vi "TempConvert.vi"(1 "All type T\nTC data \nfrom module":dbl[](array[numeric])) -> (0 "Temperature (K)":dbl[](array[numeric]))   [LabVIEW 2010]
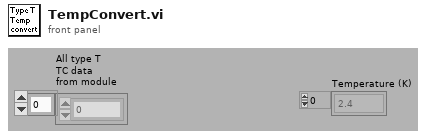
[diagram p1: front panel]
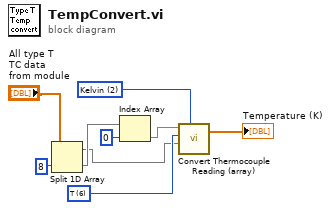
[diagram p0: block diagram]
diagram:
  w7 = u16 2 items=["Celsius", "Fahrenheit", "Kelvin", "Rankine"] ("Temperature Units (C)")
  w6 = u16 6 items=["B", "E", "J", "K", "R", "S", "T", "N", "IC (C)", "IC (F)", "Therm."] ("ThermocoupleType")
  n1 = Split 1D Array(array="All type T\nTC data \nfrom module", index=8) -> (first subarray=w3:dbl[], second subarray=w5:dbl[])
  n2 = Index Array(array=w5, index=0) -> (element=w4:dbl)
  n3 = call "Convert Thermocouple Reading (array).vi"("Temperature Units (C)"=w7, "Thermocouple Voltage"=w3, "ThermocoupleType"=w6, "Temperature"=w4) -> ("Linearized Temperature"=→"Temperature (K)":dbl[])  [unwired: 3 in]
